vi "LRS Sums (FPGA).vi"(9 "max":i32, 10 "i":i32, 11 "DataIn":i16) -> (3 "DataOut":T1)   [LabVIEW 2014]
uses:
  <vilib>/Platform/TimedLoop/XDataNode/timing_clust.ctl
  <vilib>/Platform/TimedLoop/XDataNode/nitl_modes.ctl
  <vilib>/Platform/TimedLoop/XDataNode/wakeup.ctl
  <vilib>/rvi/Emulation/niFpgaSctlEmulationGetInTimedLoop.vi
  <vilib>/rvi/Emulation/niFpgaEmulationReportErrorSimple.vi
  <vilib>/rvi/Emulation/niFpgaGetClockAttributes.vi
  <vilib>/rvi/Emulation/niFpgaCriticalErrorInLSC.vi
  <vilib>/Platform/TimedLoop/XDataNode/XDataNode.xnode
  <vilib>/rvi/FXPMathLib/FxpMul/XNode/nifxpmath_Multiplier.xnode
  <vilib>/rvi/FXPMathLib/FxpAdd/XNode/nifxpmath_Add.xnode
  <vilib>/rvi/FXPMathLib/sim/FxpSim.dll
  <vilib>/Platform/TimedLoop/XDataNode/XDNodeRunTimeDep.lvlib
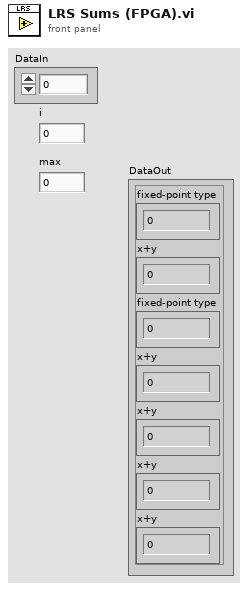
[diagram p1: front panel]
types:
  T1 = cluster{"fixed-point type":fxp<+,64,64>, "x+y":fxp<+,64,64>, "fixed-point type":fxp<+,64,64>, "x+y":fxp<+,64,64>, "x+y":fxp<+,64,64>, "x+y":fxp<+,64,64>, "x+y":fxp<+,64,64>}
  T2 = typedef "XDNodeRunTimeDep.lvlib/timing_clust.ctl" = cluster{"Expected End [f-1]":u64, "Actual End [f-1]":u64, "Finished Late? [f-1]":bool, "Expected End [i-1]":u64, "Actual End [i-1]":u64, "Finished Late? [i-1]":bool, "Expected Start [i]":u64, "Actual Start [i]":u64, "Expected Start [f]":u64, "Actual Start [f]":u64, "Source Name":string, "Structure Name":string, "Period":i64, "Deadline":i64, "Offset":i64, "Start":i64, "Priority":i32, "Timeout":i32, "Mode":T3, "Wakeup Reason":T4, "Error":errorcluster, "Source Type":string, "Secondary Source Type":string, "Global End Time":u64, "Global Start Time":u64, "Frame Duration":u64, "Iteration Duration":u64, "Assigned CPU":i32, "I/O Scan Engine Mode":u32}
  T3 = typedef "XDNodeRunTimeDep.lvlib/nitl_modes.ctl" = enum32{"No Change", "Process missed periods, maintain original phase", "Discard missed periods, maintain original phase", "Process missed periods, ignore original phase", "Discard missed periods, ignore original phase"}
  T4 = typedef "XDNodeRunTimeDep.lvlib/wakeup.ctl" = enum32{"Normal", "Aborted", "Asynchronous wakeup", "Timing source error", "Timed loop error", "Timeout"}
  T5 = cluster{"fixed-point type":fxp<+,64,64>, "x+y":fxp<+,64,64>, "fixed-point type":fxp<+,64,64>, "x+y":fxp<+,64,64>, "fixed-point type":fxp<+,64,64>, "x+y":fxp<+,64,64>, "x+y":fxp<+,64,64>}
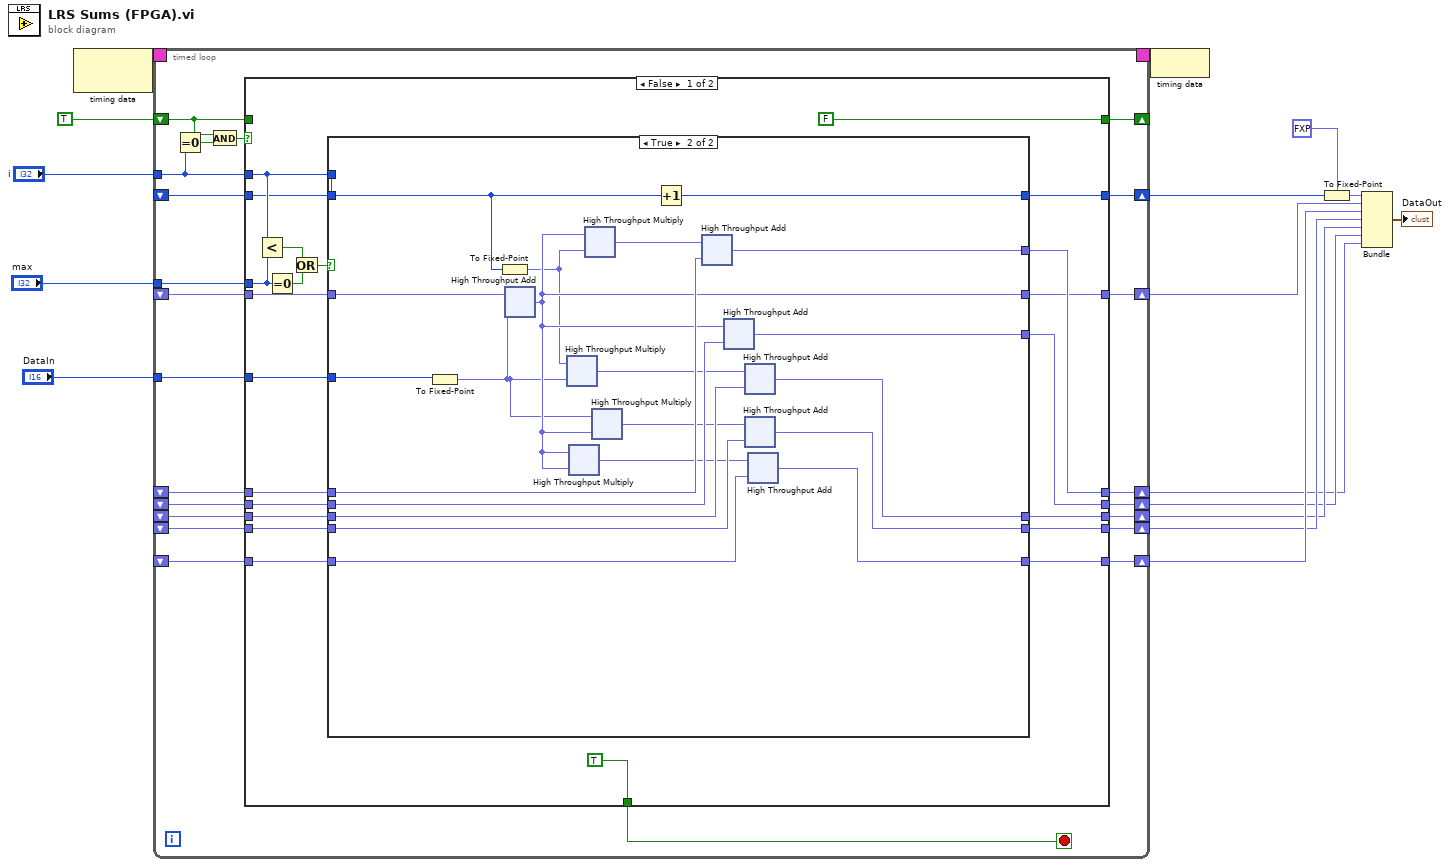
[diagram p0: block diagram]
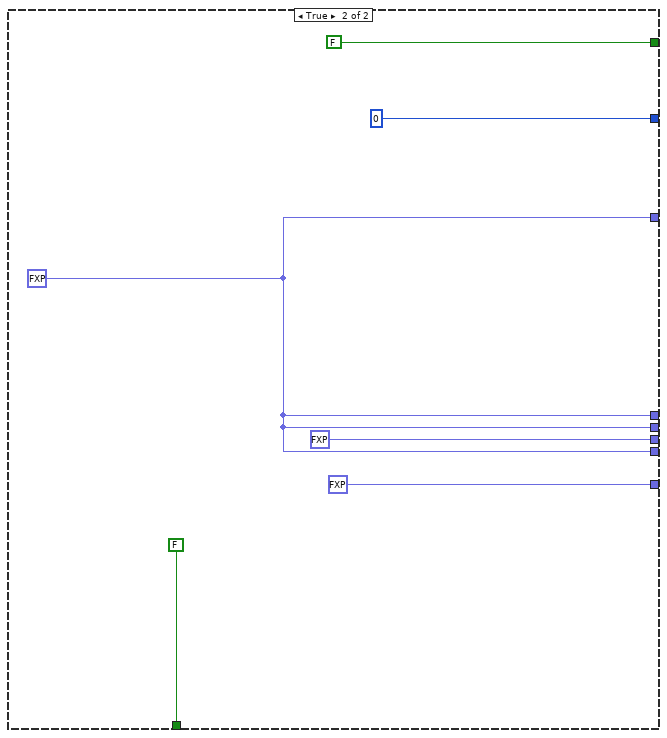
[diagram p3: hidden frame]
diagram:
  n1 = node-c288() -> (w2:T2)  [unwired: 1 in]
  n2 = timed-loop {
    shift-right: [w38] -> w15
    shift-left: _ -> [w37]
    shift-right: [w36] -> w14
    shift-left: _ -> [w35]
    shift-right: [w24] -> w13
    shift-left: _ -> [w34]
    shift-right: [w33] -> w12
    shift-left: _ -> [w32]
    shift-right: [w31] -> w11
    shift-left: _ -> [w30]
    shift-right: [w29] -> w16
    shift-left: _ -> [w28]
    tunnel: "i" -> [w21]
    shift-right: [w26] -> w6
    shift-left: _ -> [w27]
    tunnel: "max" -> [w25]
    tunnel: "DataIn" -> [w23]
    shift-right: [w20] -> _
    shift-left: TRUE -> [w18]
    timing: w2 -> [_]
    timing-out: [_] -> w1
    stop <- w22 stop-if-true
    n3 = Equal To 0?(x=w21) -> (x = 0?=w19:bool)
    n4 = And(x=w18, y=w19) -> (x .and. y?=w17:bool)
    n5 = case shown="False" w17 {
      tunnel: [w60 fxp<+,64,64> 0.0 ("fixed-point type")] -> w38
      tunnel: w37 -> [w59 _]
      tunnel: [w58 w90] -> w36
      tunnel: w35 -> [w57 _]
      tunnel: w34 -> [w56 _]
      tunnel: [w55 w90] -> w33
      tunnel: w32 -> [w54 _]
      tunnel: [w53 w90] -> w31
      tunnel: w30 -> [w52 _]
      tunnel: [w51 w90] -> w29
      tunnel: w28 -> [w50 _]
      tunnel: w21 -> [w47 _]
      tunnel: w27 -> [w45 _]
      tunnel: [w44 0] -> w26
      tunnel: w25 -> [w43 _]
      tunnel: [w42 fxp<+,64,64> 0.0 ("fixed-point type")] -> w24
      tunnel: w23 -> [w41 _]
      tunnel: [TRUE FALSE] -> w22
      tunnel: [FALSE FALSE] -> w20
      tunnel: w18 -> [_ _]
      frame False {
        n6 = Less?(x=w47, y=w43) -> (x < y?=w49:bool)
        n7 = Equal To 0?(x=w43) -> (x = 0?=w48:bool)
        n8 = Or(x=w49, y=w48) -> (x .or. y?=w46:bool)
        n9 = case shown="True" w46 {
          tunnel: [w61 w88] -> w60
          tunnel: w59 -> [w61 w87]
          tunnel: [w62 w86] -> w58
          tunnel: w57 -> [w62 w85]
          tunnel: [w63 w84] -> w42
          tunnel: w56 -> [w63 w83]
          tunnel: [w64 w82] -> w55
          tunnel: w54 -> [w64 w81]
          tunnel: [w65 w80] -> w53
          tunnel: w52 -> [w65 w79]
          tunnel: [w66 w78] -> w51
          tunnel: w50 -> [w66 w75]
          tunnel: w47 -> [_ w77]
          tunnel: w45 -> [w67 _]
          tunnel: [w67 w76] -> w44
          tunnel: w41 -> [_ w74]
          frame False {
          }
          frame True {
            n10 = To Fixed-Point(number=w74) -> (fixed-point=w73:fxp<+/-,16,16>)  [unwired: 1 in]
            n11 = To Fixed-Point(number=w77) -> (fixed-point=w72:fxp<+/-,32,32>)  [unwired: 1 in]
            n12 = xnode ("High Throughput Add")("x"=w75, "y"=w73) -> ("x+y"=w78:fxp<+,64,64>)
            n13 = xnode ("High Throughput Multiply")("x"=w72, "y"=w73) -> ("x*y"=w71:fxp<+/-,64,64>)
            n14 = xnode ("High Throughput Multiply")("x"=w78, "y"=w78) -> ("x*y"=w69:fxp<+/-,64,64>)
            n15 = xnode ("High Throughput Multiply")("x"=w78, "y"=w72) -> ("x*y"=w68:fxp<+/-,64,64>)
            n16 = xnode ("High Throughput Multiply")("x"=w73, "y"=w78) -> ("x*y"=w70:fxp<+/-,64,64>)
            n17 = Increment(x=w77) -> (x+1=w76:i32)
            n18 = xnode ("High Throughput Add")("x"=w68, "y"=w79) -> ("x+y"=w80:fxp<+,64,64>)
            n19 = xnode ("High Throughput Add")("x"=w78, "y"=w81) -> ("x+y"=w82:fxp<+,64,64>)
            n20 = xnode ("High Throughput Add")("x"=w71, "y"=w83) -> ("x+y"=w84:fxp<+,64,64>)
            n21 = xnode ("High Throughput Add")("x"=w70, "y"=w85) -> ("x+y"=w86:fxp<+,64,64>)
            n22 = xnode ("High Throughput Add")("x"=w69, "y"=w87) -> ("x+y"=w88:fxp<+,64,64>)
          }
        }
      }
      frame True {
        w90 = fxp<+,64,64> 0.0
      }
    }
  }
  n23 = node-c288(w1) -> ()
  n24 = To Fixed-Point(fixed-point type=fxp<+,64,64> 0.0, number=w6) -> (fixed-point=w5:fxp<+,64,64>)
  n25 = Bundle("fixed-point type"=w5, "x+y"=w16, "fixed-point type"=w15, "x+y"=w14, "fixed-point type"=w13, "x+y"=w12, "x+y"=w11) -> (→"DataOut":T5)  [unwired: 1 in]
